vi "LabVIEW Measurement UI - Verify Parameter Matching.vi"(0 "Measurement Client Wrapper in":refnum<class "Measurement Client Wrapper.lvclass">, 11 "error in":errorcluster) -> (4 "Measurement Client Wrapper":refnum<class "Measurement Client Wrapper.lvclass">, 6 "Status":string, 8 "Matching?":bool, 15 "error out":errorcluster)   [LabVIEW 2020, in "Measurement Client Wrapper.lvclass"]
uses:
  Measurement Client Wrapper.lvclass
  Measurement Client Wrapper.lvclass/Measurement Client Wrapper.ctl
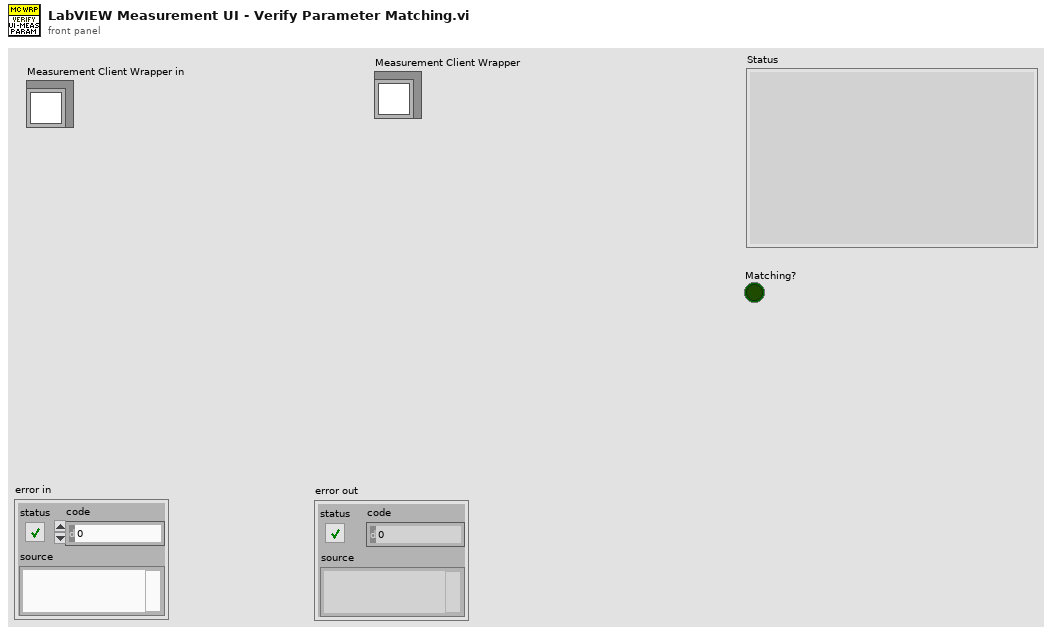
[diagram p1: front panel]
types:
  T1 = typedef "Measurement Client Wrapper.lvclass/Measurement Parameter Details.ctl" = cluster{"Name":string, "Parent":string, "ProtobufID":i32, "Measurement DataType":T2, "Array Dimension":i32}
  T2 = typedef "Measurement Client Wrapper.lvclass/Measurement DataType.ctl" = enum16{"UNSPECIFIED", "BOOL", "DOUBLE", "FLOAT", "INT32", "INT64", "STRING", "UINT32", "UINT64"}
  T3 = typedef "Measurement Client Wrapper.lvclass/Control UI MetaData.ctl" = cluster{"Name":string, "Parent":string, "LabVIEW DataType":T4, "Measurement DataType":T2, "Value":variant, "Array Dimension":i32}
  T4 = typedef "NI_Data Type.lvlib/Data Type.ctl" = enum8{"Invalid Type", "Void", "I8", "I16", "I32", "I64", "U8", "U16", "U32", "U64", "Single Float", "Double Float", "Extended Float", "Single Complex", "Double Complex", "Extended Complex", "Enum U8", "Enum U16", "Enum U32", "Enum U64", "Single Float With Unit", "Double Float With Unit", "Extended Float With Unit", "Single Complex with Unit", "Double Complex with Unit", "Extended Complex with Unit", "Boolean", "String", "Path", "Picture", "Tag", "Array", "Cluster", "Variant", "LV Variant", "Waveform", "Timestamp", "Digital Waveform", "Digital Data", "ExpressData", "Refnum", "External Data", "VI", "Poly VI", "LabVIEW Class Instance", "Fixed Point", "Set Collection", "Map Collection"}
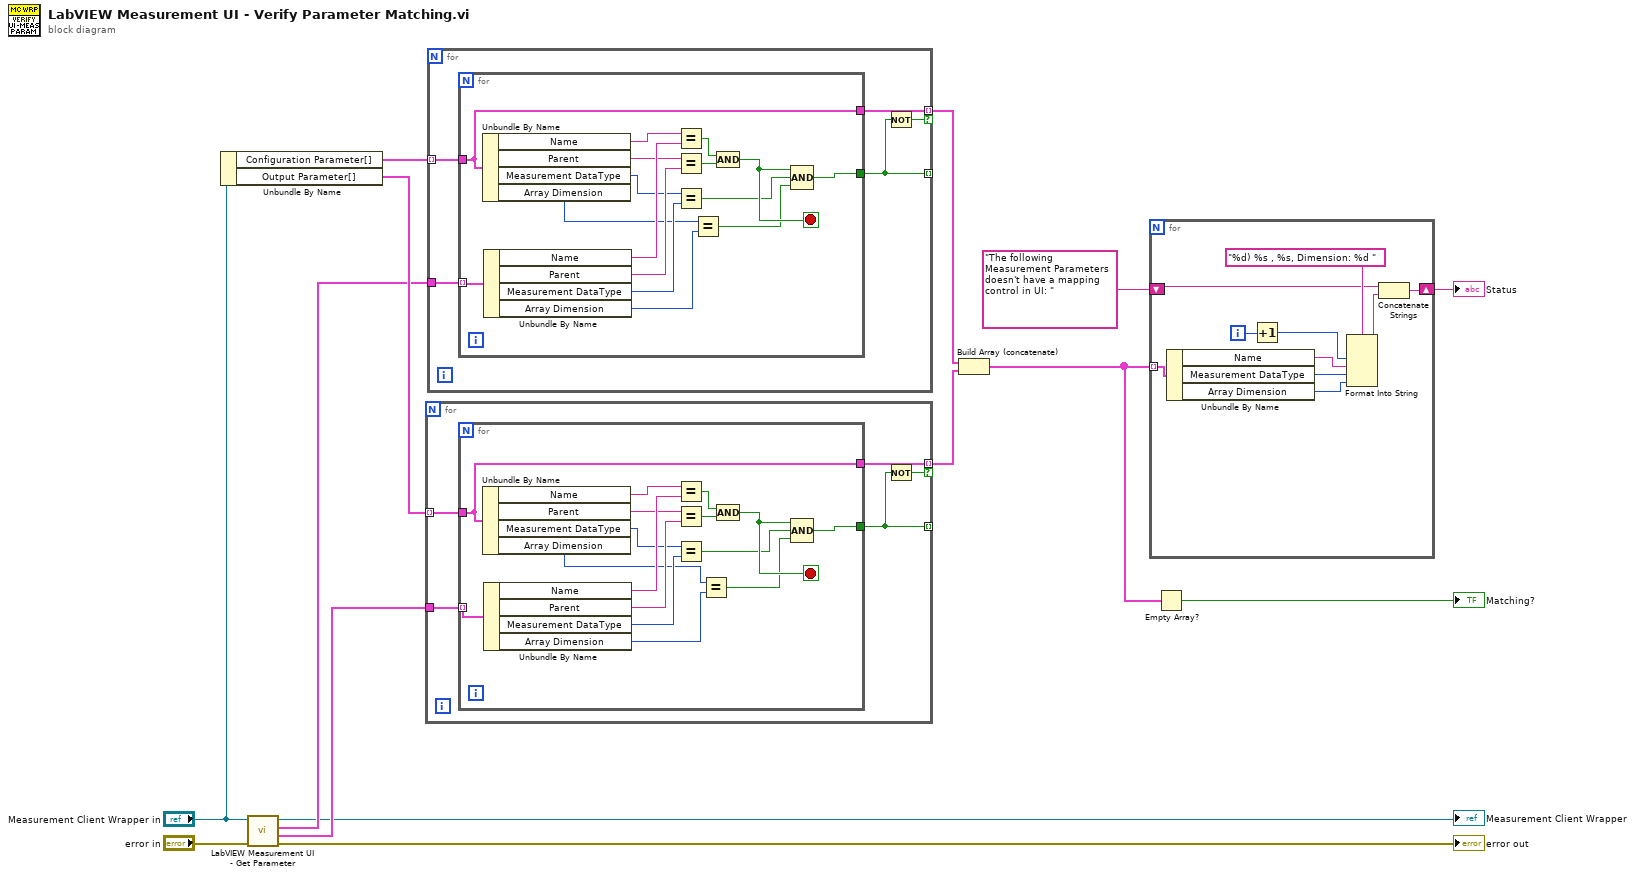
[diagram p0: block diagram]
diagram:
  n1 = Unbundle By Name("Measurement Client Wrapper in") -> ("Configuration Parameter[]"=w8:T1[], "Output Parameter[]"=w7:T1[])
  n2 = call "LabVIEW Measurement UI - Get Parameter.vi"("error in"="error in", "Measurement Client Wrapper in"="Measurement Client Wrapper in") -> ("error out"=→"error out":errorcluster, "UI Indicator Details[]"=w2:T3[], "UI Control Details[]"=w3:T3[], "Measurement Client Wrapper"=→"Measurement Client Wrapper":refnum<class "Measurement Client Wrapper.lvclass">)  [unwired: 6 in]
  n3 = for {
    tunnel: w7 -> [w18] mode=indexing
    tunnel: w2 -> [w19]
    tunnel: [w16] -> _ mode=indexing
    tunnel: [w17] -> w13 mode=indexing if=w15
    n4 = for {
      tunnel: w19 -> [w35] mode=indexing
      tunnel: [w23] -> w16
      tunnel: w18 -> [w24]
      tunnel: [w24] -> w17
      stop <- w29 stop-if-true
      n5 = Unbundle By Name(w24) -> ("Name"=w27:string, "Parent"=w26:string, "Measurement DataType"=w25:T2, "Array Dimension"=w22:i32)
      n6 = Unbundle By Name(w35) -> ("Name"=w34:string, "Parent"=w33:string, "Measurement DataType"=w32:T2, "Array Dimension"=w21:i32)
      n7 = Equal?(x=w27, y=w34) -> (x = y?=w31:bool)
      n8 = Equal?(x=w26, y=w33) -> (x = y?=w30:bool)
      n9 = Equal?(x=w25, y=w32) -> (x = y?=w28:bool)
      n10 = Equal?(x=w22, y=w21) -> (x = y?=w20:bool)
      n11 = Compound Arithmetic op=AND(w31, w30) -> (w29:bool)
      n12 = Compound Arithmetic op=AND(w29, w28, w20) -> (w23:bool)
    }
    n13 = Not(x=w16) -> (.not. x?=w15:bool)
  }
  n14 = for {
    tunnel: w8 -> [w39] mode=indexing
    tunnel: w3 -> [w40]
    tunnel: [w37] -> _ mode=indexing
    tunnel: [w38] -> w14 mode=indexing if=w36
    n15 = for {
      tunnel: w40 -> [w56] mode=indexing
      tunnel: [w44] -> w37
      tunnel: w39 -> [w45]
      tunnel: [w45] -> w38
      stop <- w50 stop-if-true
      n16 = Unbundle By Name(w45) -> ("Name"=w48:string, "Parent"=w47:string, "Measurement DataType"=w46:T2, "Array Dimension"=w43:i32)
      n17 = Unbundle By Name(w56) -> ("Name"=w55:string, "Parent"=w54:string, "Measurement DataType"=w53:T2, "Array Dimension"=w42:i32)
      n18 = Equal?(x=w48, y=w55) -> (x = y?=w52:bool)
      n19 = Equal?(x=w47, y=w54) -> (x = y?=w51:bool)
      n20 = Equal?(x=w46, y=w53) -> (x = y?=w49:bool)
      n21 = Equal?(x=w43, y=w42) -> (x = y?=w41:bool)
      n22 = Compound Arithmetic op=AND(w52, w51) -> (w50:bool)
      n23 = Compound Arithmetic op=AND(w50, w49, w41) -> (w44:bool)
    }
    n24 = Not(x=w37) -> (.not. x?=w36:bool)
  }
  n25 = Build Array (concatenate)(w14, w13) -> (w10:T1[])
  n26 = for {
    tunnel: w10 -> [w66] mode=indexing
    shift-right: [w60] -> w11
    shift-left: "The following Measurement Parameters doesn't have a mapping control in UI: " ("format string") -> [w59]
    i -> [w62]
    n27 = Unbundle By Name(w66) -> ("Name"=w63:string, "Measurement DataType"=w65:T2, "Array Dimension"=w57:i32)
    n28 = Increment(x=w62) -> (x+1=w61:i32)
    n29 = Format Into String(format string="%d) %s , %s, Dimension: %d ", w61, w63, w65, w57) -> (resulting string=w58:string)  [unwired: 2 in, 1 out]
    n30 = Concatenate Strings(w59, w58) -> (w60:string)
  }
  "Status" <- w11
  n31 = Empty Array?(array=w10) -> (empty?=→"Matching?":bool)
